vi "example_llm_chatmodel_unit_test_1.vi"() -> ()   [LabVIEW 2020]
uses:
  src/models/message_text/message_text.lvclass
  D:/Personal/LabVIEW LLMs/src/models/abstract_message_base/abstract_message_base.lvclass
  src/models/llm_openai_chatmodels/llm_openai_chatmodels.lvclass
  D:/Personal/LabVIEW LLMs/src/models/abstract_llm_base/abstract_llm_base.lvclass
  src/models/llm_azureopenai_chatmodels/llm_azureopenai_chatmodels.lvclass
  src/models/llm_anthropic_chatmodels/llm_anthropic_chatmodels.lvclass
  src/models/llm_ollama_chatmodels/llm_ollama_chatmodels.lvclass
  src/models/llm_gemini_chatmodels/llm_gemini_chatmodels.lvclass
  src/models/message_text/create_text_message.vi
  src/models/llm_openai_chatmodels/Instantiate_llm_openai.vi
  src/models/llm_azureopenai_chatmodels/Instantiate_llm_azureopenai.vi
  src/models/llm_anthropic_chatmodels/Instantiate_llm_anthropic.vi
  src/models/llm_ollama_chatmodels/Instantiate_llm_ollama.vi
  src/models/llm_gemini_chatmodels/Instantiate_llm_gemini.vi
  src/models/message_text/get_text_message_value.vi
  src/models/abstract_llm_base/abstract_llm_base.lvclass
  src/utilities/env_variables/env_variables.lvlib
  src/models/abstract_llm_chatcompletion/abstract_llm_chatcompletion.lvclass
panel:
  in  "Provider Selector":T1(tab)
  in  "model_name":string(combo)="gpt-4o-mini"
  out "openai_key":string
  in  "deployement name":string(combo)="gpt-4o-mini"
  out "azureopenai_key":string
  out "azureopenai_url":string
  out "anthropic_key":string
  in  "anthropic_model_name":string(combo)="claude-3-5-sonnet-20240620"
  in  "ollama_model_name":string(combo)="llama3.1"
  in  "Ollama URL":string="http://localhost:11434/"
  in  "model_name":string(combo)="gemini-2.0-flash"
  out "Gemini_api_key":string
  in  "temperature":dbl=1.0
  in  "Messages":cluster{"role":string, "text":string}[](array[cluster])=[{"role"="system", "text"="Act as a math teacher and guide the student in solving the problem. You should not solve the problem. Always answer in single line."}, {"role"="user", "text"="What is x in the equation 2x + 3 = 5  ?"}]
  out "error out":errorcluster
  # "1. Ensure you assign the OpenAI Key to environmental variables so it is away from the code and easy to use the examples in future.\n\n2. Use the \"Set_ENv_Var.vi\" from examples/utils folder to set the key \"labview_llm_openai_key\"."
  # "1. Ensure you assign the Azure OpenAI Key & URL to environmental variables so it is away from the code and easy to use the examples in future.\n\n2. Use the \"Set_Env_Var.vi\" from examples/utils folder to set the key \"labview_llm_azureopenai_key\" and \"labview_llm_azureopenai_url\"."
  # "1. Ensure you assign the Anthropic Key to environmental variables so it is away from the code and easy to use the examples in future.\n\n2. Use the \"Set_Env_Var.vi\" from examples/utils folder to set the key \"labview_llm_anthropic_key\"."
  # "1. Ensure you assign the Gemini API Key to environmental variables so it is away from the code and easy to use the examples in future.\n\n2. Use the \"Set_Env_Var.vi\" from examples/utils folder to set the key \"labview_llm_gemini_key\"."
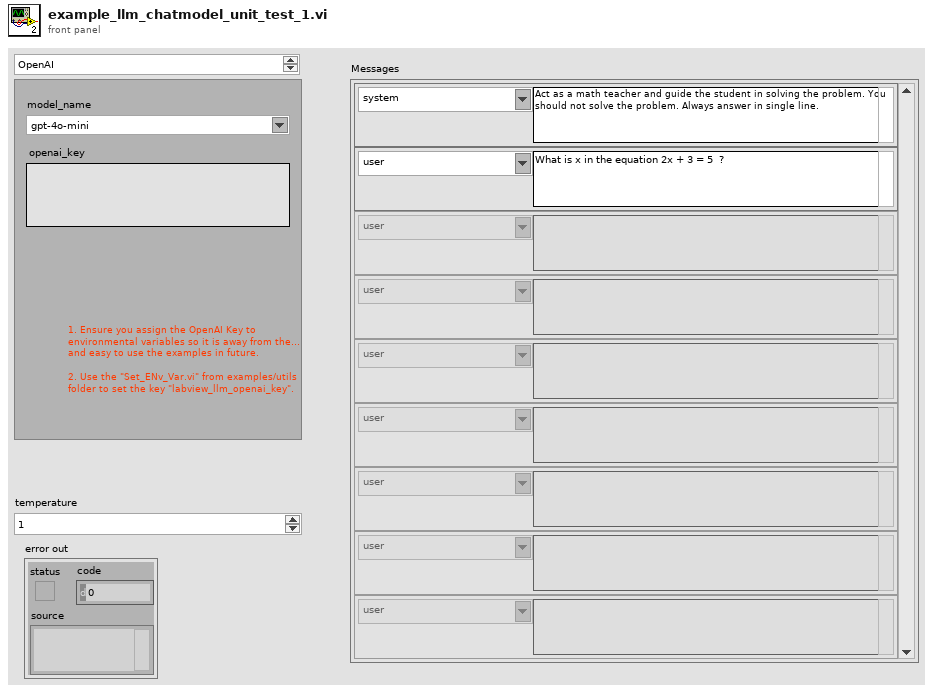
[diagram p1: front panel]
types:
  T1 = enum32{"OpenAI", "Azure OpenAI", "Anthropic", "Ollama", "Gemini"}
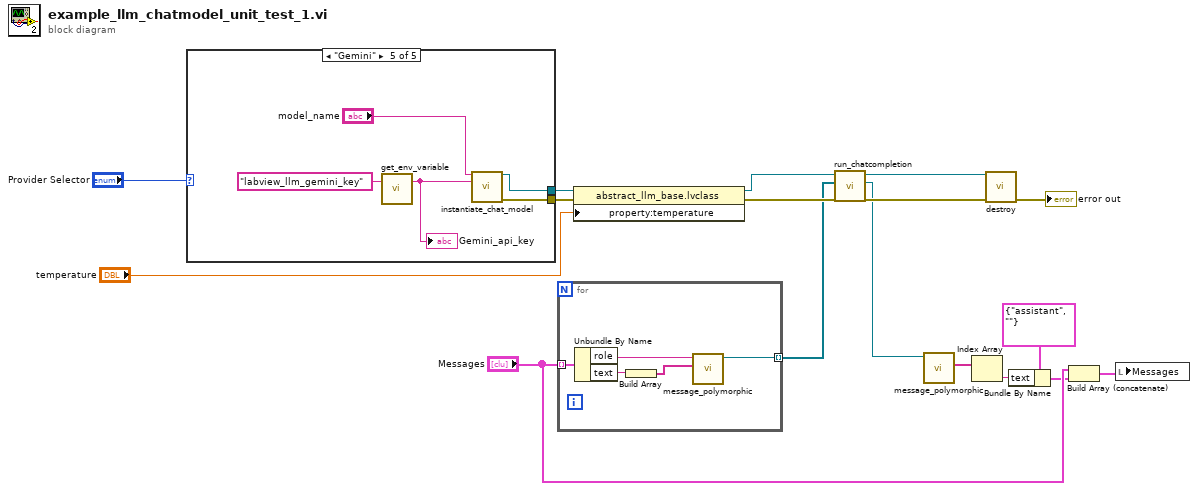
[diagram p0: block diagram]
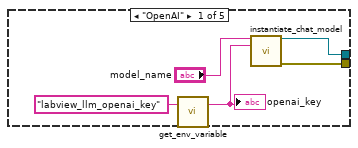
[diagram p2: hidden frame]
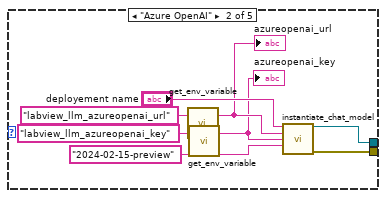
[diagram p3: hidden frame]
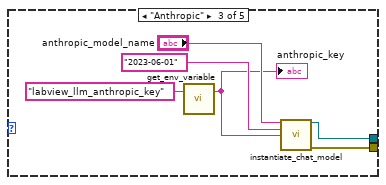
[diagram p4: hidden frame]
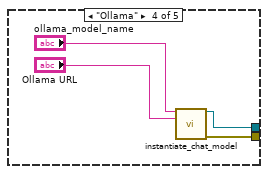
[diagram p5: hidden frame]
diagram:
  n1 = case shown="\"Gemini\"" "Provider Selector" {
    tunnel: [w21 w30 w36 w39 w44] -> w9
    tunnel: [w20 w29 w35 w40 w45] -> w7
    frame "OpenAI" {
      n2 = call "get_env_variable.vi"("Environment Variable Name"="labview_llm_openai_key") -> ("Value"=w18:string)  [unwired: 1 in, 1 out]
      "openai_key" <- w18
      n3 = call-poly "instantiate_chat_model.vi"("model_name"="model_name", "openai_key"=w18) -> ("llm_openai out"=w20:refnum<class "llm_openai_chatmodels.lvclass">, "error out"=w21:errorcluster)  [unwired: 12 in]
    }
    frame "Azure OpenAI" {
      n4 = call "get_env_variable.vi"("Environment Variable Name"="labview_llm_azureopenai_url") -> ("Value"=w25:string)  [unwired: 1 in, 1 out]
      "azureopenai_url" <- w25
      n5 = call "get_env_variable.vi"("Environment Variable Name"="labview_llm_azureopenai_key") -> ("Value"=w24:string)  [unwired: 1 in, 1 out]
      "azureopenai_key" <- w24
      n6 = call-poly "instantiate_chat_model.vi"("deployement name"="deployement name", "azure_endpoint"=w25, "azure_api_key"=w24, "api_version"="2024-02-15-preview") -> ("llm_azureopenai_chatmodels out"=w29:refnum<class "llm_azureopenai_chatmodels.lvclass">, "error out"=w30:errorcluster)  [unwired: 10 in]
    }
    frame "Anthropic" {
      n7 = call "get_env_variable.vi"("Environment Variable Name"="labview_llm_anthropic_key") -> ("Value"=w31:string)  [unwired: 1 in, 1 out]
      "anthropic_key" <- w31
      n8 = call-poly "instantiate_chat_model.vi"("model_name"="anthropic_model_name", "anthropic_version"="2023-06-01", "anthropic_key"=w31) -> ("llm_anthropic_chatmodels out"=w35:refnum<class "llm_anthropic_chatmodels.lvclass">, "error out"=w36:errorcluster)  [unwired: 11 in]
    }
    frame "Ollama" {
      n9 = call-poly "instantiate_chat_model.vi"("model_name"="ollama_model_name", "Ollama URL"="Ollama URL") -> ("llm_ollama_chatmodels out"=w40:refnum<class "llm_ollama_chatmodels.lvclass">, "error out"=w39:errorcluster)  [unwired: 12 in]
    }
    frame "Gemini" {
      n10 = call "get_env_variable.vi"("Environment Variable Name"="labview_llm_gemini_key") -> ("Value"=w41:string)  [unwired: 1 in, 1 out]
      "Gemini_api_key" <- w41
      n11 = call-poly "instantiate_chat_model.vi"("model_name"="model_name", "Gemini_api_key"=w41) -> ("llm_openai out"=w45:refnum<class "llm_gemini_chatmodels.lvclass">, "error out"=w44:errorcluster)  [unwired: 12 in]
    }
  }
  n12 = for {
    tunnel: "Messages" -> [w50] mode=indexing
    tunnel: [w46] -> w1 mode=indexing
    n13 = Unbundle By Name(w50) -> ("role"=w48:string, "text"=w49:string)
    n14 = Build Array(w49) -> (w47:string[])
    n15 = call-poly "message_polymorphic.vi"("content"=w47, "role"=w48) -> ("message_text out"=w46:refnum<class "message_text.lvclass">)  [unwired: 8 in, 1 out]
  }
  n16 = property class="abstract_llm_base.lvclass"(reference=w7, error in=w9, "property:temperature"="temperature") -> (reference out=w5:refnum<class "abstract_llm_base.lvclass">, error out=w6:errorcluster)
  n17 = call "run_chatcompletion.vi"("error in (no error)"=w6, "Messages"=w1, "abstract_llm_chatcompletion in"=w5) -> ("error out"=w3:errorcluster, "Response"=w2:refnum<class "abstract_message_base.lvclass">, "abstract_llm_chatcompletion out"=w4:refnum<class "abstract_llm_base.lvclass">)  [unwired: 6 in]
  n18 = call-poly "message_polymorphic.vi"("abstract_message_base.lvclass"=w2) -> ("content"=w10:string[])  [unwired: 8 in, 2 out]
  n19 = Index Array(array=w10) -> (element=w12:string)  [unwired: 1 in]
  n20 = call-dynamic "destroy.vi"("error in (no error)"=w3, "abstract_llm_base in"=w4) -> ("error out"=→"error out":errorcluster)  [unwired: 8 in, 1 out]
  n21 = Bundle By Name(cluster=cluster{"role":string, "text":string} {"role"="assistant", "text"=""} ("message"), "text"=w12) -> (w11:cluster{"role":string, "text":string})
  n22 = Build Array (concatenate)("Messages", w11) -> (w15:cluster{"role":string, "text":string}[])
  n23 = local write "Messages"(w15) -> ()
